vi "Configure Trigger (Periodic Timer).vi"(0 "VISA resource name":refnum<visa-resource-name>, 1 "Enable Trigger Delay (F: Disable)":bool, 2 "Trigger Level (-20 dBm)":dbl=-20.0, 5 "Sync Source (0: Off)":i32(ring) items=["Off", "External1", "External2", "RF Burst"], 7 "Period (20E-3 s)":dbl=0.02, 9 "Offset (0 s)":dbl, 11 "error in (no error)":errorcluster, 12 "Trigger Delay (1E-6 s)":dbl=1e-06, 13 "Trigger Slope (0: Positive)":i32(ring) items=["Positive", "Negative"]) -> (4 "VISA resource name out":refnum<visa-resource-name>, 15 "error out":errorcluster)   [LabVIEW 2014, in "Agilent MXA Series.lvlib"]
doc: "Configures the trigger as Periodic Timer."
uses:
  Agilent MXA Series.lvlib
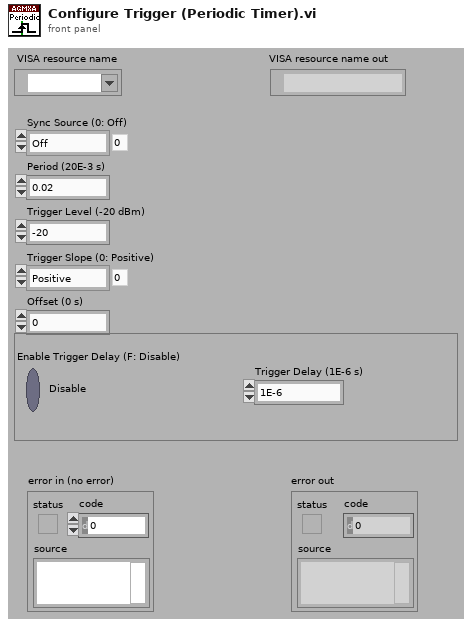
[diagram p1: front panel]
types:
  T1 = typedef "Agilent MXA Series.lvlib/Extended User Data.ctl" = cluster{"Measurement Type":i32, "Agilent MXA/EXA Model":i32}
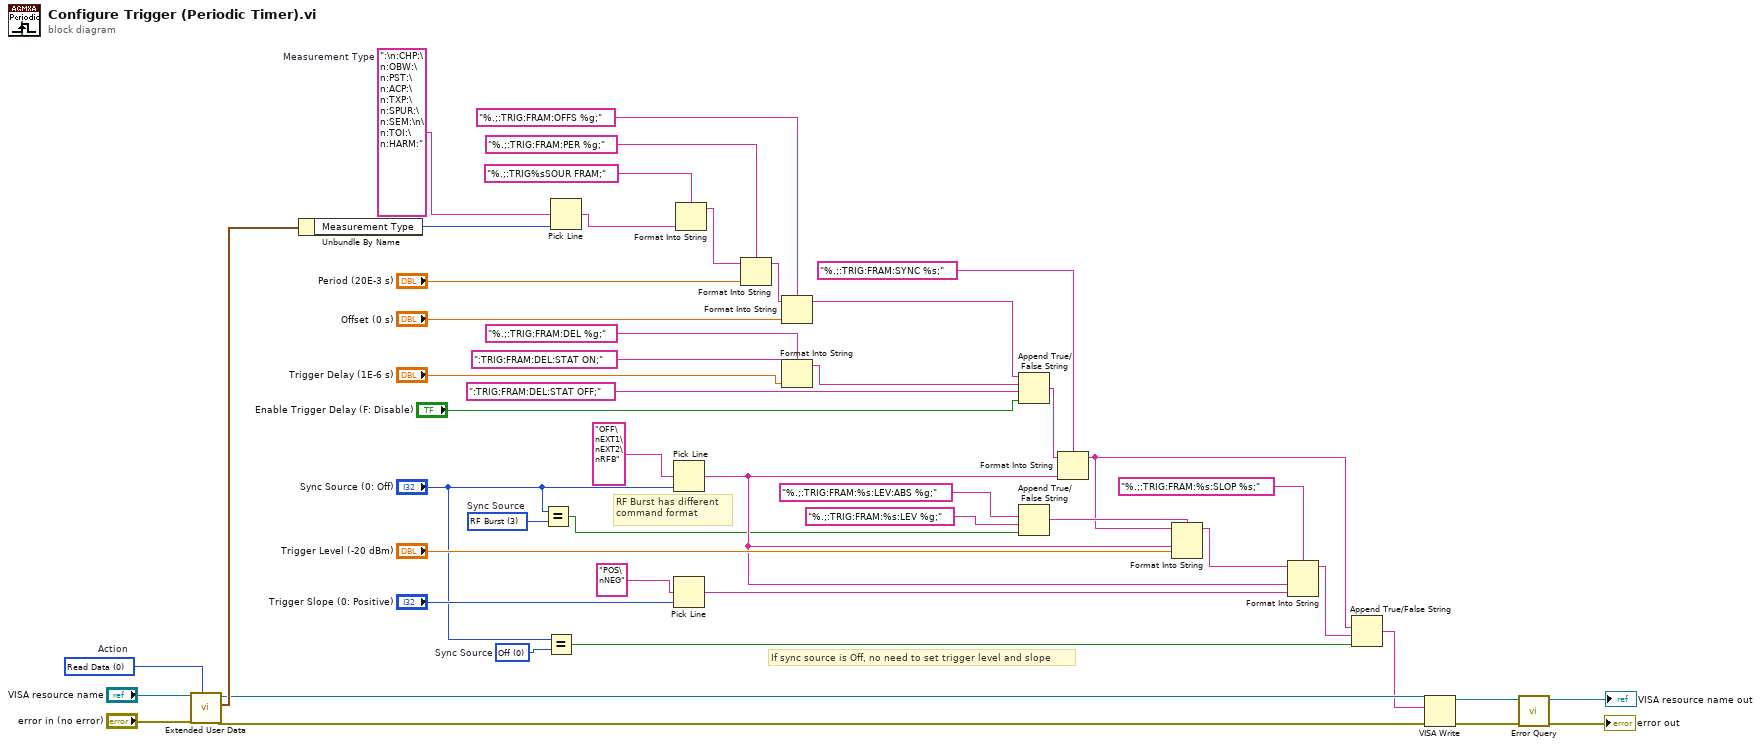
[diagram p0: block diagram]
diagram:
  w4 = 0 items=["Off", "External1", "External2", "RF Burst"]  # Sync Source
  w7 = 3 items=["Off", "External1", "External2", "RF Burst"]  # Sync Source
  w19 = 0 items=["Read Data", "Write Data", "Clear Data", "Clear ALL Data"]  # Action
  w45 = ":\n:CHP:\n:OBW:\n:PST:\n:ACP:\n:TXP:\n:SPUR:\n:SEM:\n\n:TOI:\n:HARM:"  # Measurement Type
  # "If sync source is Off, no need to set trigger level and slope"
  # "RF Burst has different \ncommand format"
  n1 = call "Extended User Data.vi"("Action (1:Write Data)"=w19, "Error In (no error)"="error in (no error)", "VISA resource name in"="VISA resource name") -> ("Error Out"=w11:errorcluster, "User Data Out"=w46:T1, "VISA resource name out"=w24:refnum<visa-resource-name>)  [unwired: 6 in]
  n2 = Unbundle By Name(w46) -> ("Measurement Type"=w44:i32)
  n3 = Equal?(x="Sync Source (0: Off)", y=w7) -> (x = y?=w6:bool)
  n4 = Equal?(x="Sync Source (0: Off)", y=w4) -> (x = y?=w3:bool)
  n5 = Pick Line(multi-line string=w45, line index=w44) -> (output string=w43:string)  [unwired: 1 in]
  n6 = Pick Line(multi-line string="OFF\nEXT1\nEXT2\nRFB", line index="Sync Source (0: Off)") -> (output string=w16:string)  [unwired: 1 in]
  n7 = Pick Line(multi-line string="POS\nNEG", line index="Trigger Slope (0: Positive)") -> (output string=w18:string)  [unwired: 1 in]
  n8 = Format Into String(format string="%.;:TRIG%sSOUR FRAM;", w43) -> (resulting string=w15:string)  [unwired: 2 in, 1 out]
  n9 = Format Into String(format string="%.;:TRIG:FRAM:PER %g;", initial string=w15, "Period (20E-3 s)") -> (resulting string=w14:string)  [unwired: 1 in, 1 out]
  n10 = Format Into String(format string="%.;:TRIG:FRAM:OFFS %g;", initial string=w14, "Offset (0 s)") -> (resulting string=w8:string)  [unwired: 1 in, 1 out]
  n11 = Format Into String(format string="%.;:TRIG:FRAM:DEL %g;", initial string=":TRIG:FRAM:DEL:STAT ON;", "Trigger Delay (1E-6 s)") -> (resulting string=w9:string)  [unwired: 1 in, 1 out]
  n12 = Append True/False String(1:"Enable Trigger Delay (F: Disable)", 2:":TRIG:FRAM:DEL:STAT OFF;" ("true string"), 3:w9, 4:w8) -> (0:w13:string)
  n13 = Append True/False String(1:w6, 2:"%.;:TRIG:FRAM:%s:LEV %g;" ("false string"), 3:"%.;:TRIG:FRAM:%s:LEV:ABS %g;" ("true string")) -> (0:w29:string)  [unwired: 1 in]
  n14 = Format Into String(format string="%.;:TRIG:FRAM:SYNC %s;", initial string=w13, w16) -> (resulting string=w2:string)  [unwired: 1 in, 1 out]
  n15 = Format Into String(format string=w29, initial string=w2, w16, "Trigger Level (-20 dBm)") -> (resulting string=w28:string)  [unwired: 1 in, 1 out]
  n16 = Format Into String(format string="%.;:TRIG:FRAM:%s:SLOP %s;", initial string=w28, w16, w18) -> (resulting string=w1:string)  [unwired: 1 in, 1 out]
  n17 = Append True/False String(1:w3, 2:w1, 3:w2) -> (0:w12:string)  [unwired: 1 in]
  n18 = VISA Write(VISA resource name=w24, write buffer=w12, error in (no error)=w11) -> (VISA resource name out=w23:refnum<visa-resource-name>, error out=w20:errorcluster)  [unwired: 1 out]
  n19 = call "Error Query.vi"("error in (no error)"=w20, "VISA resource name"=w23) -> ("error out"=→"error out":errorcluster, "VISA resource name out"=→"VISA resource name out":refnum<visa-resource-name>)  [unwired: 6 in, 2 out]
